vi "add_entry.vi"(6 "error in":errorcluster, 8 "Add-on Data":T1, 9 "Active Analog Data In":T2[](array[typedef])) -> (0 "error out":errorcluster, 3 "Active Analog Data  Out":T2[](array[typedef]))   [LabVIEW 2017]
uses:
  analog_data.ctl
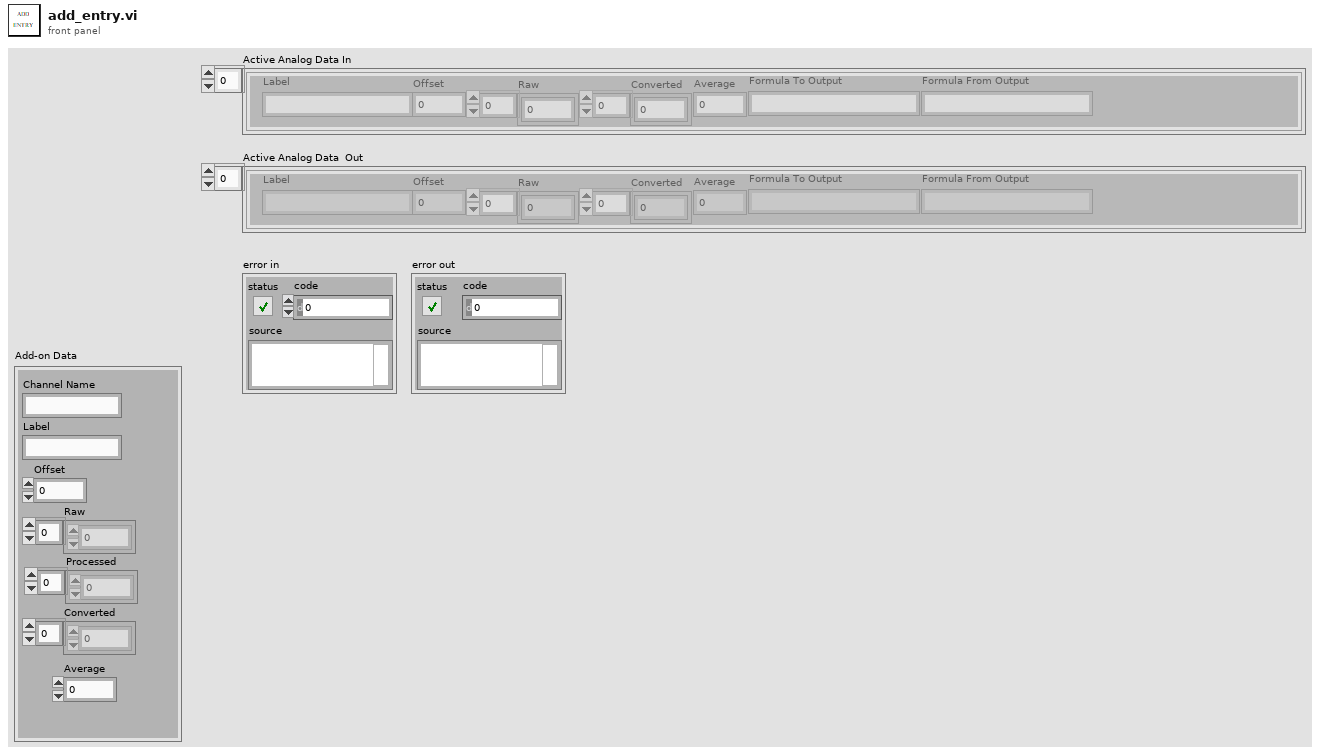
[diagram p1: front panel]
types:
  T1 = cluster{"Channel Name":string, "Label":string, "Offset":dbl, "Raw":dbl[], "Processed":dbl[], "Converted":dbl[], "Average":dbl}
  T2 = typedef "analog_data.ctl" = cluster{"Label":string, "Offset":dbl, "Raw":dbl[], "Converted":dbl[], "Average":dbl, "Formula To Output":string, "Formula From Output":string}
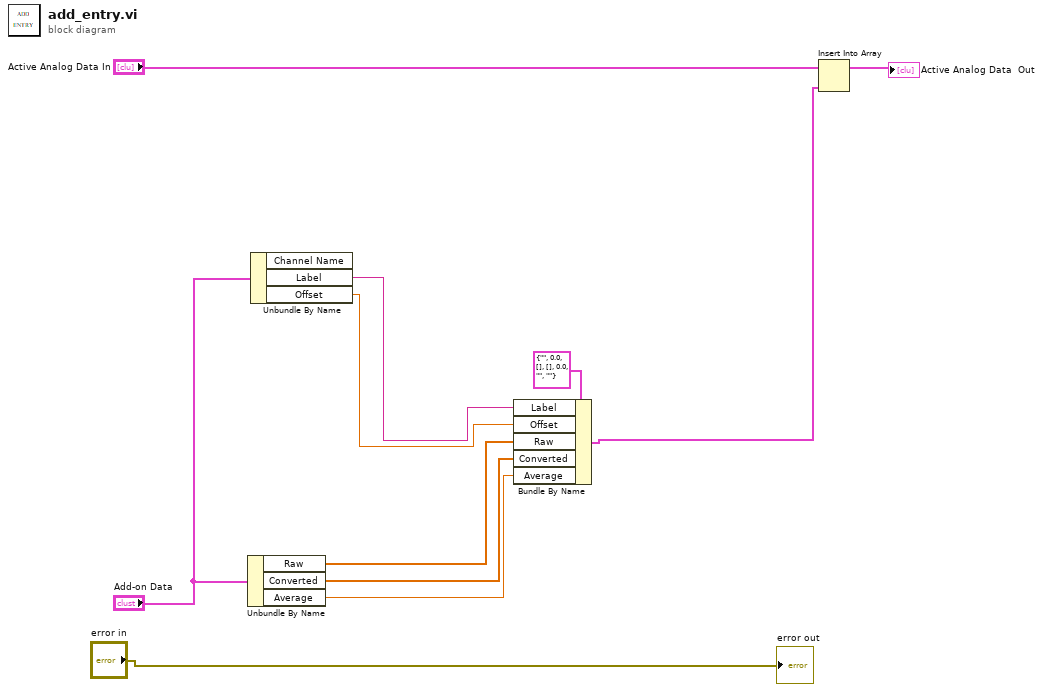
[diagram p0: block diagram]
diagram:
  n1 = Unbundle By Name("Add-on Data") -> ("Raw"=w5:dbl[], "Converted"=w4:dbl[], "Average"=w3:dbl)
  n2 = Unbundle By Name("Add-on Data") -> ("Label"=w8:string, "Offset"=w7:dbl)  [unwired: 1 out]
  n3 = Bundle By Name(cluster=T2 {"Label"="", "Offset"=0.0, "Raw"=[], "Converted"=[], "Average"=0.0, "Formula To Output"="", "Formula From Output"=""} ("Analog Data"), "Label"=w8, "Offset"=w7, "Raw"=w5, "Converted"=w4, "Average"=w3) -> (w1:T2)
  n4 = Insert Into Array(array="Active Analog Data In", new element=w1) -> (→"Active Analog Data  Out":T2[])  [unwired: 1 in]
  "error out" <- "error in"
